vi "Target Analyze.vi"(0 "Original Image_in":T3, 1 "Color Plane":i32(ring) items=["Red", "Green", "Blue", "Hue", "Saturation", "Luminance", "Value", "Intensity"], 3 "Range":cluster{"Lower value":sgl, "Upper value":sgl}={"Lower value"=150.0, "Upper value"=255.0} {"Lower value" scale=0.0..255.0; "Upper value" scale=0.0..255.0}, 4 "Camera Type":enum16{"206", "1011"}(ring)=enum."1011", 5 "Annotate":bool=TRUE, 6 "Target Choice":i8(knob) scale=0.0..2.0, 7 "Mask":T3, 9 "gray":T3) -> (10 "Numeric Target Info (X,Y,D)":dbl[](array[numeric]), 11 "Target corners pixels":T2(array[cluster]), 12 "Target Info":T4(array[cluster]), 13 "Targert Found":bool, 14 "Original Image_out+":T3(plugin-control), 15 "Processed Image":T3(plugin-control), 16 "Position of Target Center Y":dbl, 17 "Distance [m]":dbl, 18 "Position of Target Center X":dbl, 19 "Particle Scores":T1)   [LabVIEW 2012]
doc: "This VI demonstrates how to do target processing on a laptop computer. It uses the same MJPG VI as the dashboard, sets a few of the important camera properties that impact processing, and carries out the same processing steps as the RT example also included in this project."
uses:
  <vilib>/vision/Image Controls.llb/IMAQ Image.ctl
  <vilib>/vision/NI_Vision_Development_Module.lvlib
panel:
  out "Center Target":bool
  in  "Area Size Limit %":dbl=0.5
  in  "Particle Count Limit":i32=10
  in  "Score Limits":T5={"Rect Coverage"=60.0, "X Edge Strength"=40.0, "Y Edge Strength"=60.0, "Center"=75.0, "Outer"=75.0}
  in  "Processing":enum32{"Monochrome", "Color"}(tab)
  out "Value":cluster{i32, i32}
  out "Saturation":cluster{i32, i32}
  in  "Value":i32=255
  in  "Saturation":i32=255
  in  "Hue":i32(knob)=65 scale=0.0..255.0
  in  "Margins":cluster{"Hue":i32, "Sat":i32, "Val":i32}={"Hue"=33, "Sat"=53, "Val"=9} {"Sat" scale=0.0..80.0; "Val" scale=0.0..80.0; "Hue" scale=0.0..80.0}
  out "Hue":cluster{i32, i32}
  # "Information:\nProcessing can be based on color or light intensity.\nParticles within the image are scored by rectangle coverage, aspect ratio, and\nedge strength/hollowness. A particle is considered a target if all scores\nare above the score limits you set. Particles can be annotated -- surrounded by\na rectangle and scores drawn to the left .\nTo control the number of particles being scored, use the count limit and the size\nlimit.\nBe sure to set the Camera IP before running. The distance calculation uses the\ncamera type to index the value of the lens view angle."
  # "Click in the image to choose  color for processing."
  # "Green scores are above the limit, orange are below. Inner/outer rect\nindicates all passed."
  # "Lower/Upper"
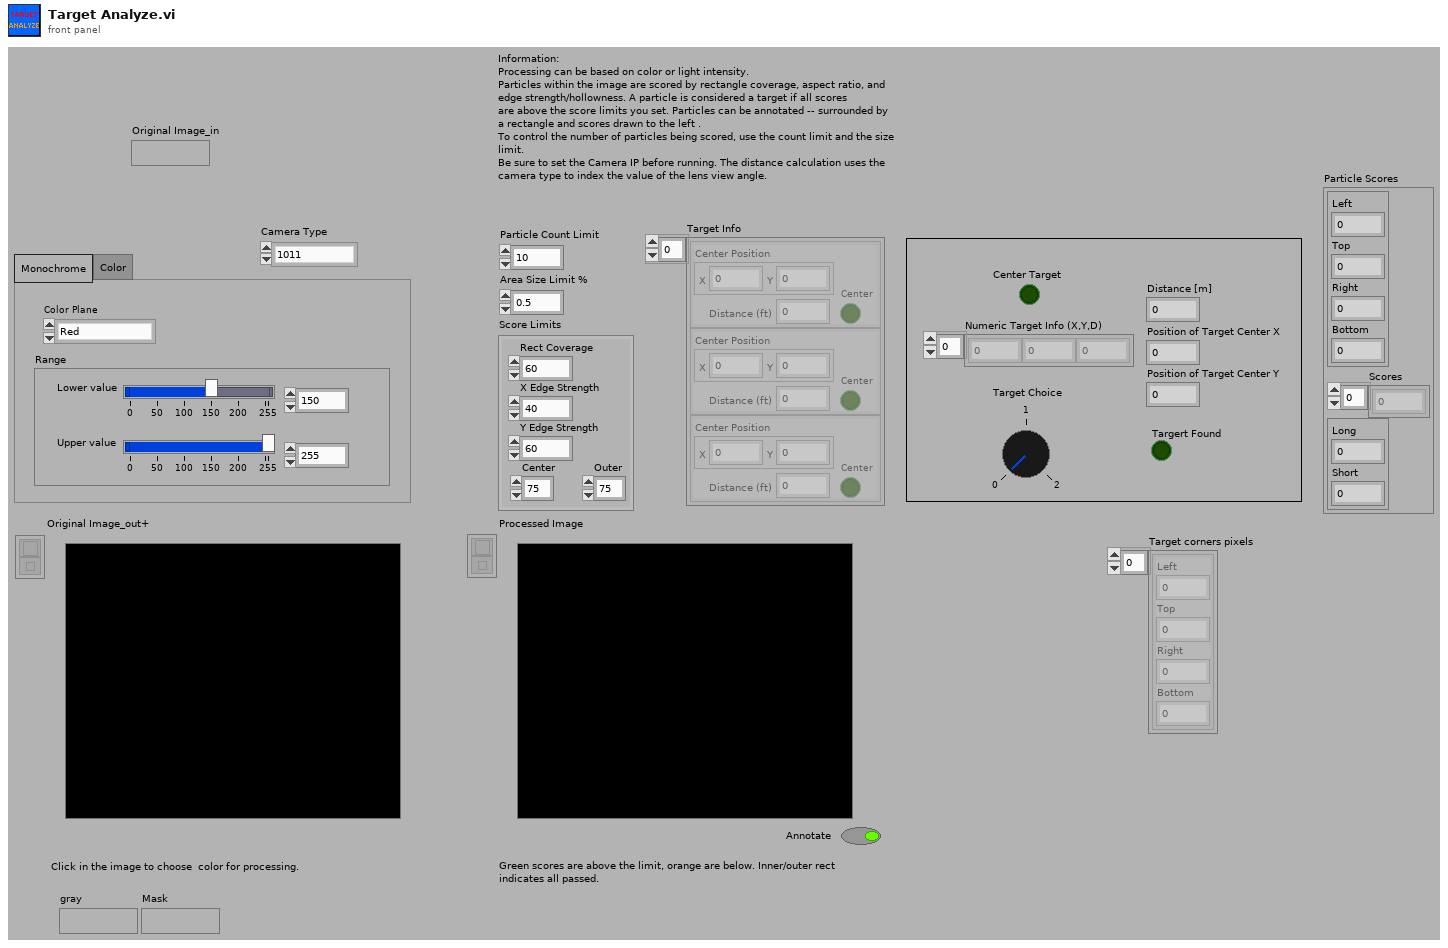
[diagram p1: front panel]
types:
  T1 = cluster{cluster{"Left":dbl, "Top":dbl, "Right":dbl, "Bottom":dbl}, "Scores":dbl[], cluster{"Long":dbl, "Short":dbl}}
  T2 = cluster{"Left":dbl, "Top":dbl, "Right":dbl, "Bottom":dbl}[]
  T3 = typedef "IMAQ Image.ctl" = refnum<image>
  T4 = cluster{"Center Position":cluster{"X":dbl, "Y":dbl}, "Distance (ft)":dbl, "Center":bool}[]
  T5 = cluster{"Rect Coverage":dbl, "X Edge Strength":dbl, "Y Edge Strength":dbl, "Center":dbl, "Outer":dbl}
  T6 = cluster{"Position":cluster{"X":dbl, "Y":dbl}, "Distance (ft)":dbl, "Center Target":bool}[]
  T7 = typedef "Image Type" = u32
  T8 = cluster{cluster{"Left":dbl, "Top":dbl, "Right":dbl, "Bottom":dbl}, "Scores":dbl[], cluster{"Long":dbl, "Short":dbl}}[]
  T9 = cluster{"Target Center (-1 to 1)":cluster{"X":dbl, "Y":dbl}, "Distance (ft)":dbl, "Center Target":bool}
  T10 = cluster{"Target Center (-1 to 1)":cluster{"X":dbl, "Y":dbl}, "Distance (ft)":dbl, "Center Target":bool}[]
  T11 = cluster{"Left":dbl, "Top":dbl, "Right":dbl, "Bottom":dbl}
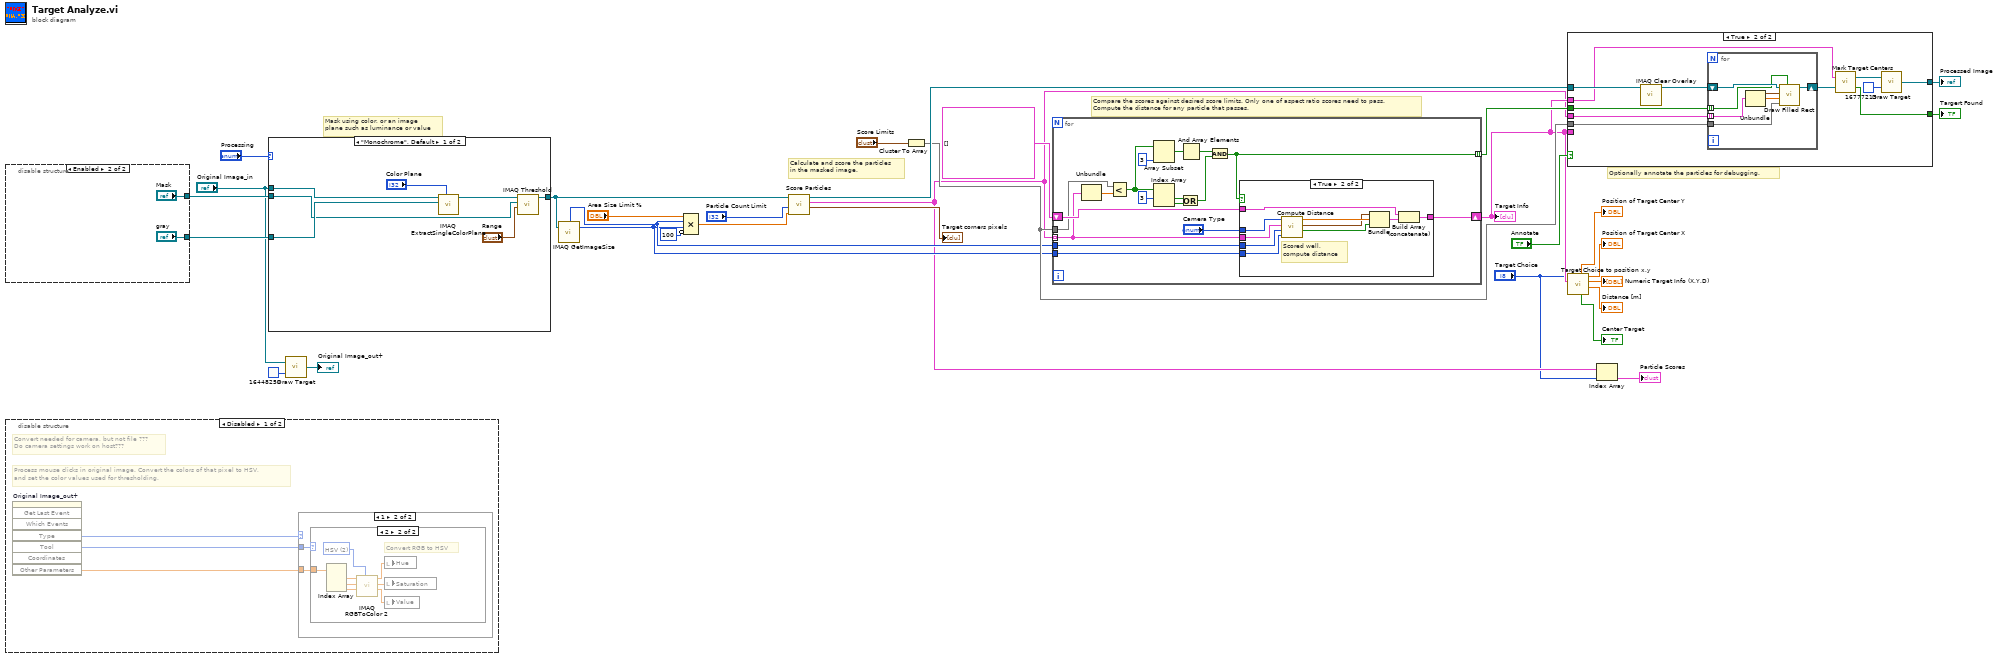
[diagram p0: block diagram]
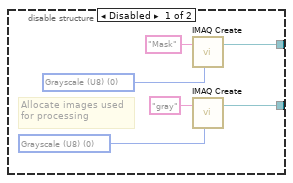
[diagram p2: hidden frame]
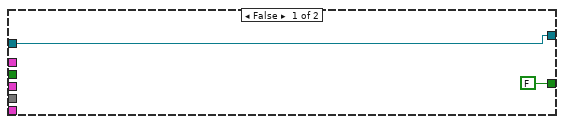
[diagram p6: hidden frame]
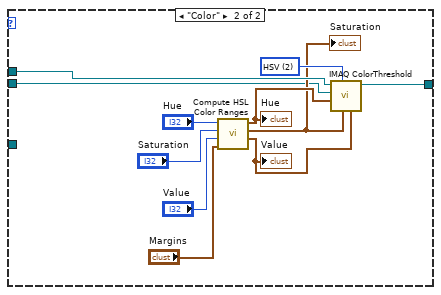
[diagram p7: hidden frame]
diagram:
  # "Optionally annotate the particles for debugging."
  # "Compare the scores against desired score limits. Only one of aspect ratio scores need to pass.\nCompute the distance for any particle that passes."
  # "Calculate and score the particles\nin the masked image."
  # "Mask using color, or an image\nplane such as luminance or value"
  n1 = disable-structure shown="Enabled" {
    disable-tunnel: [w35 "gray"] -> w31
    disable-tunnel: [w32 "Mask"] -> w30
    frame Disabled {
      w33 = T7 0 items=["Grayscale (U8)", "Grayscale (I16)", "Grayscale (SGL)", "Complex (CSG)", "RGB (U32)", "HSL (U32)", "RGB (U64)", "Grayscale (U16)"] ("Image Type")
      w37 = T7 0 items=["Grayscale (U8)", "Grayscale (I16)", "Grayscale (SGL)", "Complex (CSG)", "RGB (U32)", "HSL (U32)", "RGB (U64)", "Grayscale (U16)"] ("Image Type")
      # "Allocate images used\nfor processing"
      n2 = call "IMAQ Create"("Image Name"="Mask", "Image Type"=w33) -> ("New Image"=w32:T3)  [unwired: 2 in, 2 out]
      n3 = call "IMAQ Create"("Image Name"="gray", "Image Type"=w37) -> ("New Image"=w35:T3)  [unwired: 2 in, 2 out]
    }
    frame Enabled {
    }
  }
  n4 = disable-structure shown="Disabled" {
    frame Disabled {
      # "Process mouse clicks in original image. Convert the colors of that pixel to HSV,\nand set the color values used for thresholding."
      # "Convert needed for camera, but not file ???\nDo camera settings work on host???"
      n5 = invoke on="Original Image_out+" class="ImageControl" method="Get Last Event"() -> ("Type"=w40:i32, "Tool"=w41:i32, "Other Parameters"=w42:sgl[])  [unwired: 8 in, 5 out]
      n6 = case shown="1" w40 {
        tunnel: w41 -> [_ w44]
        tunnel: w42 -> [_ w43]
        frame 0, Default {
        }
        frame 1 {
          n7 = case shown="2" w44 {
            tunnel: w43 -> [_ w52]
            frame Default {
            }
            frame 2 {
              w51 = u16 2 items=["RGB", "HSL", "HSV", "HSI", "CIE L*a*b*", "CIE XYZ"] ("Color Mode")
              # "Convert RGB to HSV"
              n8 = Index Array(array=w52) -> (element #1=w50:sgl, element #2=w48:sgl, element #3=w46:sgl)  [unwired: 3 in]
              n9 = call "IMAQ RGBToColor 2"("Color Mode"=w51, "Blue value"=w46, "Green value"=w48, "Red value"=w50) -> ("Blue or Luma or Val or Inten or Z or b*value"=w45:dbl, "Green or Sat or Y or a* value"=w47:dbl, "Red or Hue or X or L* value"=w49:dbl)  [unwired: 4 in, 1 out]
              n10 = local write "Hue"(w49) -> ()
              n11 = local write "Saturation"(w47) -> ()
              n12 = local write "Value"(w45) -> ()
            }
          }
        }
      }
    }
    frame Enabled {
    }
  }
  n13 = case shown="\"Monochrome\", Default" "Processing" {
    tunnel: "Original Image_in" -> [w59 w70]
    tunnel: w31 -> [w58 _]
    tunnel: [w55 w69] -> w24
    tunnel: w30 -> [w53 w60]
    frame "Monochrome", Default {
      n14 = call "IMAQ ExtractSingleColorPlane"("Color Plane"="Color Plane", "Image Dst"=w58, "Image Src"=w59) -> ("Image Dst Out"=w57:T3)  [unwired: 1 in, 7 out]
      n15 = call "IMAQ Threshold"("Range"="Range", "Image Dst"=w53, "Image Src"=w57) -> ("Image Dst Out"=w55:T3)  [unwired: 3 in, 5 out]
    }
    frame "Color" {
      w68 = u16 2 items=["RGB", "HSL", "HSV", "HSI"] ("Color Mode")
      n16 = call "Compute HSL Color Ranges.vi"("Margins"="Margins", "Luminance"="Value", "Saturation"="Saturation", "Hue"="Hue") -> ("Lum Range"=w61:cluster{i32, i32}, "Sat Range"=w62:cluster{i32, i32}, "Hue Range"=w67:cluster{i32, i32})  [unwired: 5 in]
      "Hue" <- w67
      "Saturation" <- w62
      "Value" <- w61
      n17 = call "IMAQ ColorThreshold"("Blue or Luma or Val or Inten Range"=w61, "Green or Sat Range"=w62, "Color Mode"=w68, "Red or Hue Range"=w67, "Image Dst"=w60, "Image Src"=w70) -> ("Image Dst Out"=w69:T3)  [unwired: 4 in, 1 out]
    }
  }
  n18 = call "Draw Target.vi"("Color"=u32 16448250, "Original Image"="Original Image_in") -> ("Image Out"=→"Original Image_out+":T3)
  n19 = call "IMAQ GetImageSize"("Image"=w24) -> ("Y Resolution"=w18:i32, "X Resolution"=w19:i32)  [unwired: 3 in, 1 out]
  n20 = Compound Arithmetic op=MULTIPLY("Area Size Limit %", w19, w18, invert 100 ("value")) -> (w17:dbl)
  n21 = call "Score Particles.vi"("Area Size Limit"=w17, "Particle Count Limit"="Particle Count Limit", "Image Refnum in"=w24) -> ("Target corners pixels"=→"Target corners pixels":T2, "Scored Particle Info"=w3:T8, "Image Refnum out"=w28:T3)  [unwired: 6 in]
  n22 = Cluster To Array(cluster="Score Limits") -> (array=w22:dbl[])
  n23 = for {
    shift-right: [w86] -> w10
    shift-left: T6 [] -> [w87]
    tunnel: w19 -> [w85]
    tunnel: w3 -> [w71] mode=indexing
    tunnel: w22 -> [w83]
    tunnel: w18 -> [w82]
    tunnel: [w73] -> w21 mode=indexing
    n24 = Unbundle(w71) -> ("Scores"=w84:dbl[])  [unwired: 2 out]
    n25 = Less?(x=w83, y=w84) -> (x < y?=w79:bool[])
    n26 = Array Subset(array=w79, length=3) -> (w80:bool[])  [unwired: 1 in]
    n27 = Index Array(array=w79, index #1=3 ("length")) -> (element #1=w77:bool, element #2=w76:bool)  [unwired: 1 in]
    n28 = Or(x=w77, y=w76) -> (x .or. y?=w75:bool)
    n29 = And Array Elements(Boolean array=w80) -> (logical AND=w74:bool)
    n30 = And(x=w74, y=w75) -> (x .and. y?=w73:bool)
    n31 = case shown="True" w73 {
      tunnel: w87 -> [w88 w98]
      tunnel: [w88 w97] -> w86
      tunnel: w85 -> [_ w96]
      tunnel: "Camera Type" -> [_ w94]
      tunnel: w82 -> [_ w92]
      tunnel: w71 -> [_ w91]
      frame False {
        # "Didn't score well enough"
      }
      frame True {
        # "Scored well,\ncompute distance"
        n32 = call "Compute Distance.vi"("Y Image Resolution"=w92, "X Image Resolution"=w96, "Particle Scores"=w91, "Camera Type"=w94) -> ("Center Target"=w90:bool, "Target Center (-1 to 1)"=w93:cluster{"X":dbl, "Y":dbl}, "Distance (ft)"=w95:dbl)  [unwired: 5 in]
        n33 = Bundle("Target Center (-1 to 1)"=w93, "Distance (ft)"=w95, "Center Target"=w90) -> (w89:T9)  [unwired: 1 in]
        n34 = Build Array (concatenate)(w98, w89) -> (w97:T10)
      }
    }
  }
  "Target Info" <- w10
  n35 = case shown="True" "Annotate" {
    tunnel: w28 -> [w100 w111]
    tunnel: [w100 w101] -> w26
    tunnel: w3 -> [_ w107]
    tunnel: w22 -> [_ w109]
    tunnel: w21 -> [_ w108]
    tunnel: w10 -> [_ _]
    tunnel: [FALSE ("Target") w106] -> w11
    tunnel: w10 -> [_ w105]
    frame False {
    }
    frame True {
      n36 = call "IMAQ Clear Overlay"("Image"=w111) -> ("Image Out"=w110:T3)  [unwired: 2 in, 8 out]
      n37 = for {
        shift-right: [w112] -> w103
        shift-left: w110 -> [w118]
        tunnel: w107 -> [w113] mode=indexing
        tunnel: w109 -> [w115]
        tunnel: w108 -> [w114] mode=indexing
        n38 = Unbundle(w113) -> (w116:T11, "Scores"=w117:dbl[])  [unwired: 1 out]
        n39 = call "Draw Filled Rect.vi"("Limit Passed"=w114, "Limits"=w115, "Scores"=w117, "Bounding Box"=w116, "image in"=w118) -> ("image out"=w112:T3)  [unwired: 6 in]
      }
      n40 = call "Mark Target Centers.vi"("Processed Image"=w103, "Target Info"=w105) -> ("Target"=w106:bool, "Image Out"=w102:T3)
      n41 = call "Draw Target.vi"("Color"=u32 16777215, "Original Image"=w102) -> ("Image Out"=w101:T3)
    }
  }
  "Processed Image" <- w26
  "Targert Found" <- w11
  n42 = call "Target Choice to position x,y.vi"("Array"=w10, "Target Choice"="Target Choice") -> ("Distance [m]"=→"Distance [m]":dbl, "Numeric Target Info (X,Y,D)"=→"Numeric Target Info (X,Y,D)":dbl[], "Position of Target Center X"=→"Position of Target Center X":dbl, "Center Target"=→"Center Target":bool, "Position of Target Center Y"=→"Position of Target Center Y":dbl)  [unwired: 5 in]
  n43 = Index Array(array=w3, index="Target Choice") -> (element=→"Particle Scores":T1)
